vi "Producto Comprado.vi"(8 "error in (no error)":errorcluster, 10 "Cluster Producto":T1, 11 "UI Actor in":refnum<class "UI Actor.lvclass">) -> (0 "error out":errorcluster, 3 "UI Actor out":refnum<class "UI Actor.lvclass">)   [LabVIEW 2019, in "UI Actor.lvlib" / "UI Actor.lvclass"]
uses:
  UI Actor.lvclass
  UI Actor.lvclass/UI Actor.ctl
  USD Actor Messages/Precio VS Credito Msg/Precio VS Credito Msg.lvclass/Precio VS Credito Msg.ctl
  <vilib>/ActorFramework/Message Enqueuer/Message Enqueuer.lvclass/Message Enqueuer.ctl
  MXN Actor Messages/Precio VS Credito Msg/Precio VS Credito Msg.lvclass/Precio VS Credito Msg.ctl
  <vilib>/ActorFramework/Message Enqueuer/Enqueue.vi
  USD Actor Messages/Precio VS Credito Msg/Precio VS Credito Msg.lvclass
  C:/Program Files (x86)/National Instruments/LabVIEW 2019/vi.lib/ActorFramework/Message/Message.lvclass
  MXN Actor Messages/Precio VS Credito Msg/Precio VS Credito Msg.lvclass
  <vilib>/ActorFramework/Message Priority Queue/Priority Enqueue.vi
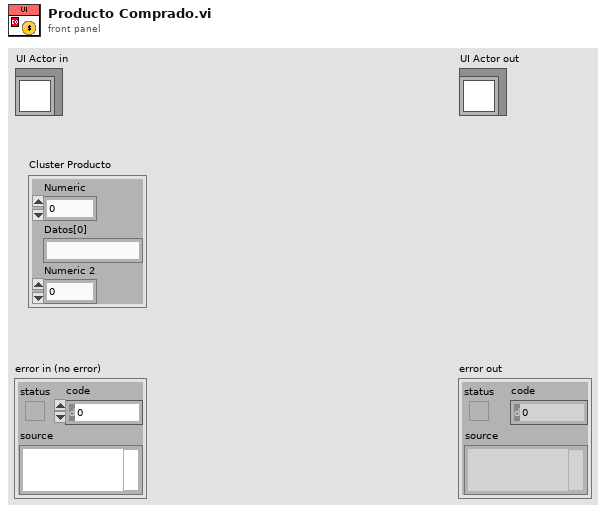
[diagram p1: front panel]
types:
  T1 = cluster{"Numeric":i32, "Datos[0]":string, "Numeric 2":dbl}
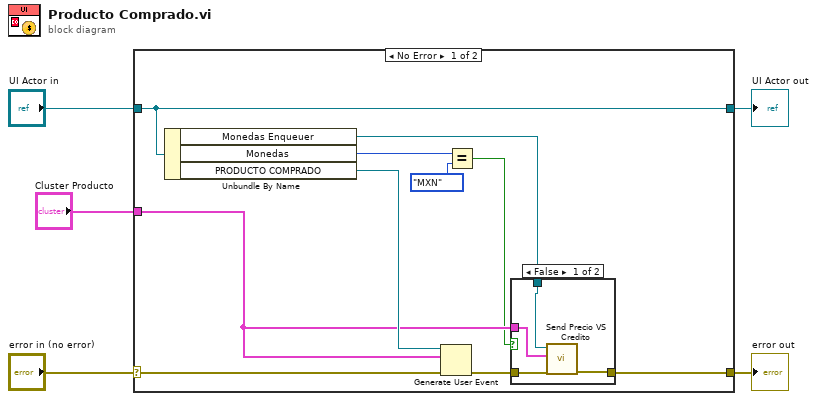
[diagram p0: block diagram]
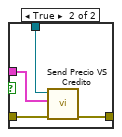
[diagram p2: hidden frame]
diagram:
  n1 = case shown="No Error" "error in (no error)" {
    selector: "error in (no error)" -> [w14 w25]
    tunnel: [w11 w25] -> w4
    tunnel: [w15 w24] -> w2
    tunnel: "UI Actor in" -> [w15 w24]
    tunnel: "Cluster Producto" -> [w9 _]
    frame No Error {
      n2 = Unbundle By Name(w15) -> ("Monedas Enqueuer"=w10:refnum<class "Message Enqueuer.lvclass">, "Monedas"=w8:enum16{"MXN", "USD"}, "PRODUCTO COMPRADO"=w13:refnum<user-event>)
      n3 = Generate User Event(user event=w13, event data cluster=w9, error in=w14) -> (error out=w12:errorcluster)  [unwired: 1 in, 1 out]
      n4 = Equal?(x=w8, y=enum16{"MXN", "USD"}."MXN") -> (x = y?=w6:bool)
      n5 = case shown="False" w6 {
        tunnel: w12 -> [w19 w23]
        tunnel: [w18 w22] -> w11
        tunnel: w10 -> [w16 w21]
        tunnel: w9 -> [w17 w20]
        frame False {
          n6 = call "Send Precio VS Credito.vi"("error in (no error)"=w19, "Cluster Producto"=w17, "Message Enqueuer"=w16) -> ("error out"=w18:errorcluster)  [unwired: 7 in, 1 out]
        }
        frame True {
          n7 = call "Send Precio VS Credito.vi"("error in (no error)"=w23, "Cluster Producto"=w20, "Message Enqueuer"=w21) -> ("error out"=w22:errorcluster)  [unwired: 7 in, 1 out]
        }
      }
    }
    frame Error {
    }
  }
  "error out" <- w4
  "UI Actor out" <- w2
